vi "ClassAttributes_ReadClassAttributes_4x4x4.vi"(8 "error in (no error)":errorcluster, 11 "reference in":refnum<class>) -> (0 "error out":errorcluster, 3 "reference out":refnum<class>)   [LabVIEW 2020]
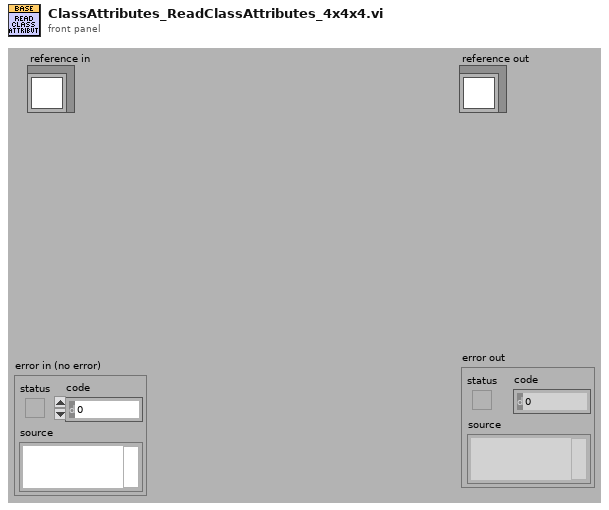
[diagram p1: front panel]
types:
  T1 = typedef "ClassAttributes_ClassAttributes.ctl" = cluster{"classAttribute1":bool}
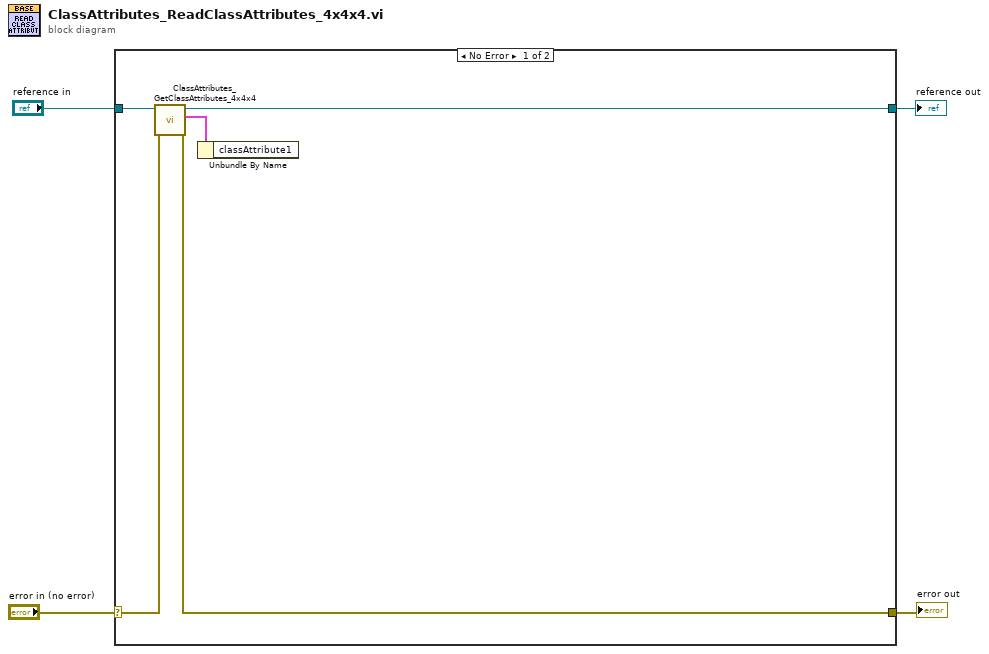
[diagram p0: block diagram]
diagram:
  n1 = case shown="No Error" "error in (no error)" {
    selector: "error in (no error)" -> [w9 w11]
    tunnel: [w7 w11] -> w3
    tunnel: [w5 w10] -> w1
    tunnel: "reference in" -> [w6 w10]
    frame No Error {
      n2 = call <resource>:"ClassAttributes_GetClassAttributes_4x4x4.vi"("error in (no error)"=w9, "reference in"=w6) -> ("error out"=w7:errorcluster, "Class attribute"=w8:T1, "reference out"=w5:refnum<class>)  [unwired: 6 in, 1 out]
      n3 = Unbundle By Name(w8) -> ()  [unwired: 1 out]
    }
    frame Error {
    }
  }
  "error out" <- w3
  "reference out" <- w1
